vi "Write Voltage.vi"(8 "error in":errorcluster, 10 "Voltage":dbl, 11 "69X_79X in":refnum<class "7976A.lvclass">) -> (0 "error out":errorcluster, 3 "69X_79X out":refnum<class "7976A.lvclass">)   [LabVIEW 2019, in "7976A.lvlib" / "7976A.lvclass"]
uses:
  Library/7976A.lvclass
  builds/Instruments/PowerSupply.lvlibp/Library/PowerSupply.lvclass
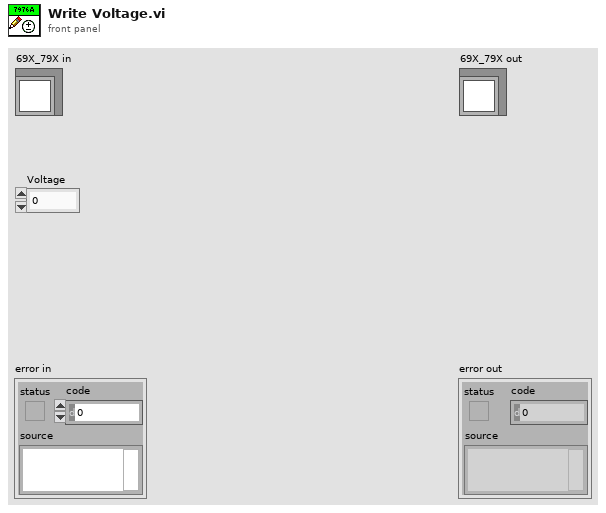
[diagram p1: front panel]
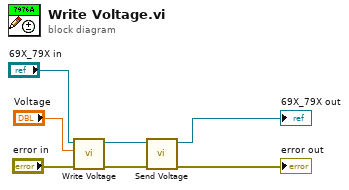
[diagram p0: block diagram]
diagram:
  n1 = call-parent "Write Voltage.vi"("error in"="error in", "Voltage"="Voltage", "PowerSupply in"="69X_79X in") -> ("error out"=w3:errorcluster, "PowerSupply out"=w4:refnum<class "7976A.lvclass">)  [unwired: 7 in]
  n2 = call "Send Voltage.vi"("error in"=w3, "69X_79X in"=w4) -> ("error out"=→"error out":errorcluster, "69X_79X out"=→"69X_79X out":refnum<class "7976A.lvclass">)  [unwired: 8 in]
